vi "CommonVIs_CloseControlRefs.vi"(0 "Event Registration Refnum":refnum<event-registration>, 1 "ControlRefs":refnum<vi>[](array[refnum]), 2 "error in (no error)":errorcluster) -> (16 "error out":errorcluster)   [LabVIEW 2020]
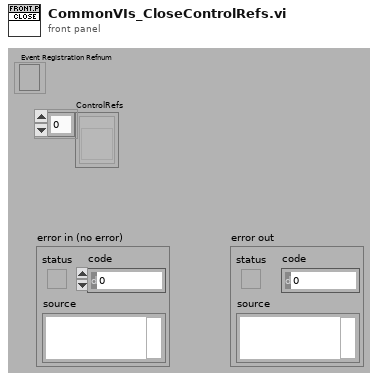
[diagram p1: front panel]
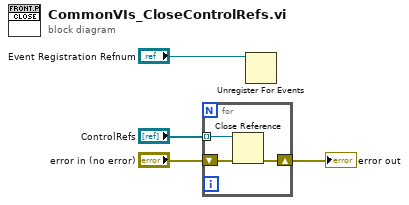
[diagram p0: block diagram]
diagram:
  n1 = for {
    shift-right: [w5] -> w2
    shift-left: "error in (no error)" -> [w7]
    tunnel: "ControlRefs" -> [w6] mode=indexing
    n2 = Close Reference(reference=w6, error in (no error)=w7) -> (error out=w5:errorcluster)
  }
  "error out" <- w2
  n3 = Unregister For Events(event registration refnum="Event Registration Refnum") -> ()  [unwired: 1 in, 1 out]
